vi "Queue Remove.vi"(6 "timeout(ms: -1)":i32=-1, 8 "error in (no error)":errorcluster, 11 "queue name":string) -> (0 "error out":errorcluster, 1 "timeout？":bool, 2 "data":variant, 3 "event":string)   [LabVIEW 2020]
uses:
  Control/Queue Data.ctl
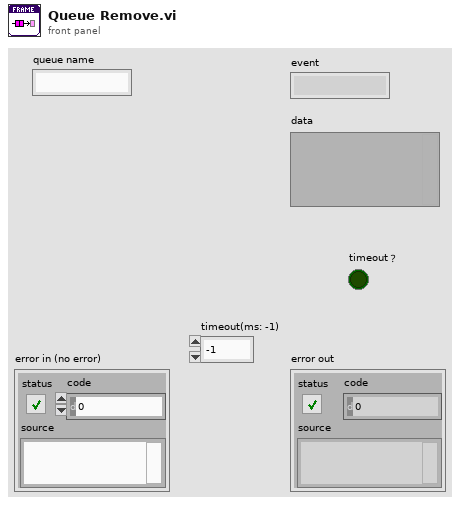
[diagram p1: front panel]
types:
  T1 = typedef "Queue Data.ctl" = cluster{"event":string, "data":variant}
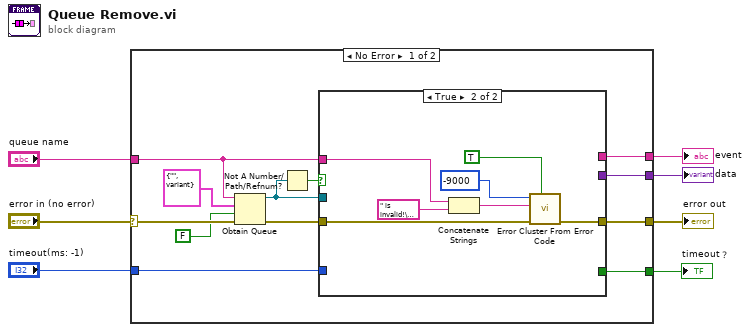
[diagram p0: block diagram]
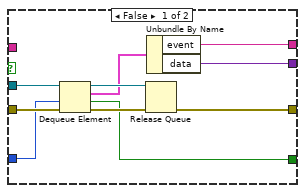
[diagram p2: hidden frame]
diagram:
  n1 = case shown="No Error" "error in (no error)" {
    selector: "error in (no error)" -> [w19 w37]
    tunnel: [w13 w37] -> w6
    tunnel: "queue name" -> [w14 _]
    tunnel: "timeout(ms: -1)" -> [w11 _]
    tunnel: [w10 _] -> w3
    tunnel: [w9 _] -> w2
    tunnel: [w8 _] -> w1
    frame No Error {
      n2 = Obtain Queue(name (unnamed)=w14, element data type=T1 {"event"="", "data"=variant} ("Cluster"), create if not found? (T)=FALSE, error in (no error)=w19) -> (queue out=w12:refnum<queue>, error out=w16:errorcluster)  [unwired: 1 in, 1 out]
      n3 = Not A Number/Path/Refnum?(number/path/refnum=w12) -> (NaN/Path/Refnum?=w15:bool)
      n4 = case shown="True" w15 {
        tunnel: w16 -> [w29 w32]
        tunnel: w14 -> [_ w31]
        tunnel: [w23 w30] -> w13
        tunnel: w12 -> [w28 _]
        tunnel: w11 -> [w27 _]
        tunnel: [w22 _] -> w9
        tunnel: [w21 _] -> w10
        tunnel: [w20 _] -> w8
        frame False {
          n5 = Dequeue Element(queue=w28, timeout in ms (-1)=w27, error in (no error)=w29) -> (queue out=w26:refnum<queue>, element=w24:T1, timed out?=w20:bool, error out=w25:errorcluster)
          n6 = Release Queue(queue=w26, error in (no error)=w25) -> (error out=w23:errorcluster)  [unwired: 1 in, 2 out]
          n7 = Unbundle By Name(w24) -> ("event"=w21:string, "data"=w22:variant)
        }
        frame True {
          n8 = Concatenate Strings(w31, " is invalid!\nEnsure the queue has been created!" ("字符串")) -> (w34:string)
          n9 = call <vilib>:"Error Cluster From Error Code.vi"("show call chain? (False)"=TRUE, "error in (no error)"=w32, "error message (\"\")"=w34, "error code (0)"=-9000) -> ("error out"=w30:errorcluster)  [unwired: 5 in]
        }
      }
    }
    frame Error {
    }
  }
  "error out" <- w6
  "event" <- w3
  "data" <- w2
  "timeout？" <- w1
